vi "mcs6atest.vi"() -> ()   [LabVIEW 2016]
panel:
  out "CHN Status":T1 {"Dummy" format="%.2f"; "Starts" format="%.2f"; "Sweeps" format="%.2f"; "Roirate" format="%.2f"; "RoiSum" format="%.2f"; "TotalSum" format="%.2f"; "Fifo full" format="%.2f"; "Runtime" format="%.2f"}
  in  "Spectrum #":i32
  out "Settings":T2 {"dummy3" format="%.2f"; "dummy2" format="%.2f"; "bitshift" format="%.0x"; "Active" format="%.0x"; "Offset" format="%.0x"; "Param" format="%.0x"; "dummy1" format="%.2f"; "Roipreset" format="%.2f"; "cftfak" format="%.0x"}
  out "MCSADat Error":i32
  out "Data":u32[](graph)
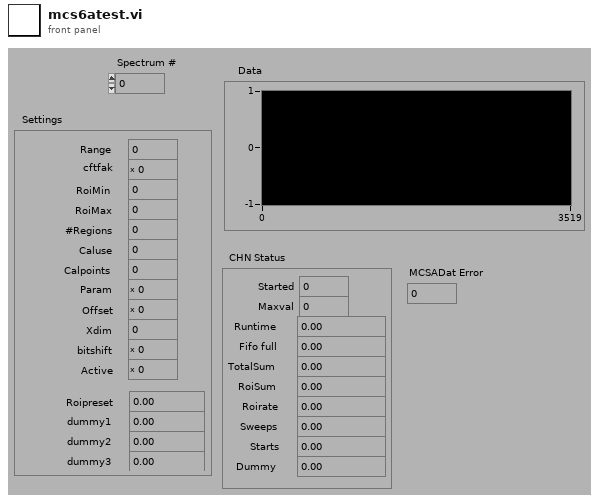
[diagram p1: front panel]
types:
  T1 = cluster{"Started":i32, "Maxval":u32, "Runtime":dbl, "Fifo full":dbl, "TotalSum":dbl, "RoiSum":dbl, "Roirate":dbl, "Sweeps":dbl, "Starts":dbl, "Dummy":dbl}
  T2 = cluster{"Range":i32, "cftfak":i32, "RoiMin":i32, "RoiMax":i32, "#Regions":i32, "Caluse":i32, "Calpoints":i32, "Param":i32, "Offset":i32, "Xdim":i32, "bitshift":i32, "Active":i32, "Roipreset":dbl, "dummy1":dbl, "dummy2":dbl, "dummy3":dbl}
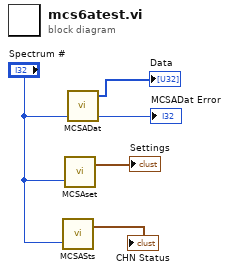
[diagram p0: block diagram]
diagram:
  n1 = call "MCSASts.vi"("CHN #"="Spectrum #") -> ("CHN Status"=→"CHN Status":T1)  [unwired: 1 in, 1 out]
  n2 = call "MCSAset.vi"("Spect #"="Spectrum #") -> ("Settings"=→"Settings":T2)  [unwired: 1 in, 1 out]
  n3 = call "MCSADat.vi"("Spectrum #"="Spectrum #") -> ("MCSADat Error"=→"MCSADat Error":i32, "Data"=→"Data":u32[])  [unwired: 2 in, 1 out]
